vi "SC10_get_shutter_state2.vi"(8 "error in (no error)":errorcluster, 11 "VISA resource name":refnum<visa-resource-name>) -> (0 "error out":errorcluster, 1 "number":i32, 2 "open(true)":bool, 3 "VISA resource name out":refnum<visa-resource-name>)   [LabVIEW 2010]
panel:
  out "substring":string
  out "read buffer":string
  out "return count 2":u32
  out "return count":u32
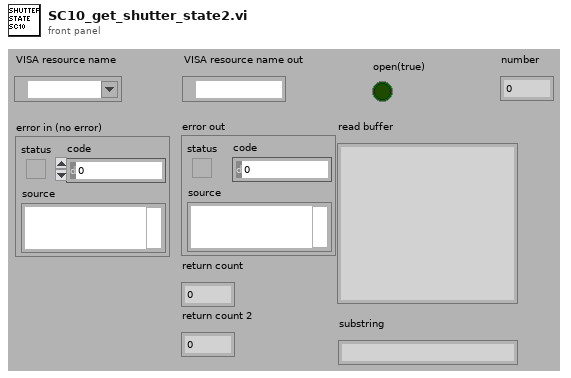
[diagram p1: front panel]
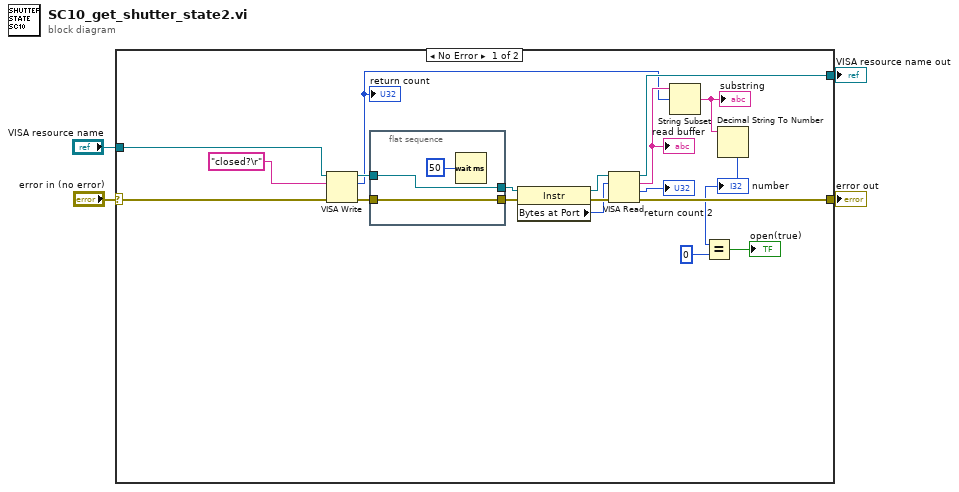
[diagram p0: block diagram]
diagram:
  n1 = case shown="No Error" "error in (no error)" {
    selector: "error in (no error)" -> [w21 w27]
    tunnel: [w20 w27] -> w3
    tunnel: [w18 w28] -> w2
    tunnel: "VISA resource name" -> [w17 w28]
    frame No Error {
      n2 = VISA Write(VISA resource name=w17, write buffer="closed?\r", error in (no error)=w21) -> (VISA resource name out=w23:refnum<visa-resource-name>, return count=w15:u32, error out=w22:errorcluster)
      "return count" <- w15
      n3 = flat-sequence {
        tunnel: w23 -> [w25]
        tunnel: [w25] -> w12
        tunnel: w22 -> [w24]
        tunnel: [w24] -> w11
        frame #0 {
          n4 = Wait (ms)(milliseconds to wait=u32 50) -> ()  [unwired: 1 out]
        }
      }
      n5 = property class="Instr"(reference=w12, error in=w11) -> (reference out=w13:refnum<visa-resource-name>, error out=w14:errorcluster, "Bytes at Port"=w10:u32)
      n6 = VISA Read(VISA resource name=w13, byte count=w10, error in (no error)=w14) -> (VISA resource name out=w18:refnum<visa-resource-name>, read buffer=w16:string, return count=→"return count 2":u32, error out=w20:errorcluster)
      "read buffer" <- w16
      n7 = String Subset(string=w16, offset (0)=w15) -> (substring=w8:string)  [unwired: 1 in]
      "substring" <- w8
      n8 = Decimal String To Number(string=w8) -> (number=w7:i32)  [unwired: 2 in, 1 out]
      "number" <- w7
      n9 = Equal?(x=w7, y=0) -> (x = y?=→"open(true)":bool)
    }
    frame Error {
    }
  }
  "error out" <- w3
  "VISA resource name out" <- w2
